vi "EHLRequest.vi"(6 "Reply":T1, 9 "Message Data":variant, 11 "Message Queue in":refnum<class "ModuleQueue.lvclass">) -> (0 "error out":errorcluster)   [LabVIEW 2024, in "AddNewEvent.lvlib"]
uses:
  AddNewEvent.lvlib
  RQMHCore/Shared/ModuleShared.lvlib
  RQMHCore/ModuleCore/Reply.ctl
  RQMHCore/ModuleCore/Module.lvclass
  RQMHCore/ModQueue/ModuleQueue.lvclass
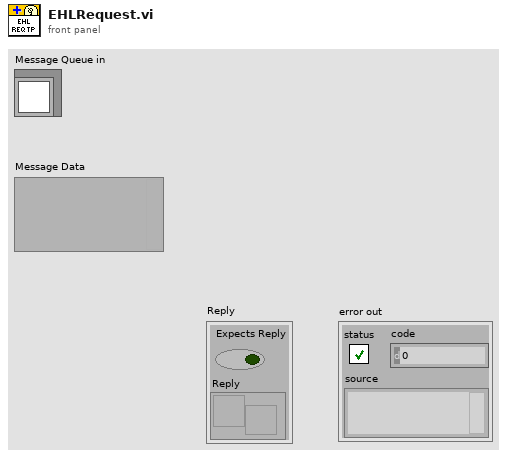
[diagram p1: front panel]
types:
  T1 = typedef "Module.lvclass/Reply.ctl" = cluster{"Expects Reply":bool, "Reply":refnum<notifier>}
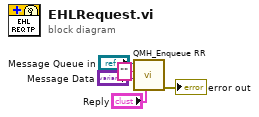
[diagram p0: block diagram]
diagram:
  n1 = call "QMH_Enqueue RR.vi"("Reply"="Reply", "Message Data"="Message Data", "Message"="", "Message Queue in"="Message Queue in") -> ("error out"=→"error out":errorcluster)  [unwired: 6 in, 1 out]
